vi "AskUserForModules.vi"(4 "MultiModule":bool, 6 "SkipDialog":bool, 7 "SPCModulesArray":T2[](array[typedef]) {"Bus Number" min=-1 max=255 step=1; "Base I/O Addr" format="%.0x"; "Init Status" min=-10 max=0 step=1; "in Use" min=-1 max=1 step=1; "Slot Number" min=-1 max=255 step=1; "Module Type" items=["SPC-600"=600, "SPC-630"=630, "SPC-700"=700, "SPC-730"=730, "SPC-130"=130, "SPC-830"=830, "SPC-140"=140, "SPC-930"=930, "DPC-230"=230, "SPC-150"=150, "SPC-150 N"=151, "SPC-150 NX"=152, "SPC-130 EM"=131, "SPC-130 EMN"=132, "SPC-130IN"=135, "SPC-130INX"=136, "SPC-130INXX"=137, "SPC-160"=160, "SPC-160 X"=161, "SPC-160 PCIE"=162, "SPC-180 N"=180, "SPC-180 NX"=181, "SPC-180 NXX"=182, "SPC-180 N-USB"=185, "SPC-180 NX-USB"=186, "SPC-180 NXX-USB"=187, "SPC-QC-104"=104, "SPC-QC-004"=4, "SPC-QC-106"=106, "DPC-330"=330, "PMS-800"=800, "SPC-590"=590, "Simulation"=-1]}, 8 "Error In":errorcluster={"Status"=FALSE, "Code"=0, "Source"="no error"}, 9 "Serial Number":string[](array[string]), 10 "ModuleNoArray":i16[](array[numeric]), 11 "DLL Path":path=path "C:/Program Files (x86)/BH/SPCM/DLL/spcm64.dll") -> (0 "Error Out":errorcluster, 1 "ActiveSerialNumbers":string[](array[string]), 2 "ModuleListboxStrings":string[][](array[string]), 3 "DLL Path":path=path "C:/Program Files (x86)/BH/SPCM/DLL/spcm64.dll", 5 "ActiveModuleNo":i16[](array[numeric]))   [LabVIEW 2023]
doc: "This VI presents the user with a dialog displaying all available modules with type and serial number information.\nOne or several modules can be chosen to continue with the application flow.\nThe dialog can be skipped if only one module is present or the choice already known.\nThe input values are provided by the Initialize.vi.\n\ninfo@becker-hickl.com"
uses:
  SPC_Wrappers/SPC_Controls/SPCModInfo.ctl
  SPC_Wrappers/SPC_Controls/ModuleType.ctl
panel:
  in  "Active":T1
  out "ActiveNameOfModules":string[](array[string])
  out "Module Type":string[](array[string])
  out "Name of Modules":string[](array[string])
  in  "OK":bool
  in  "Activate All":bool
  in  "Frame":string
  # "Please Choose Your TCSPC Module(s)"
  # "Developer: Frank Quadt, M.sc\n\n42 is the answer for everything!"
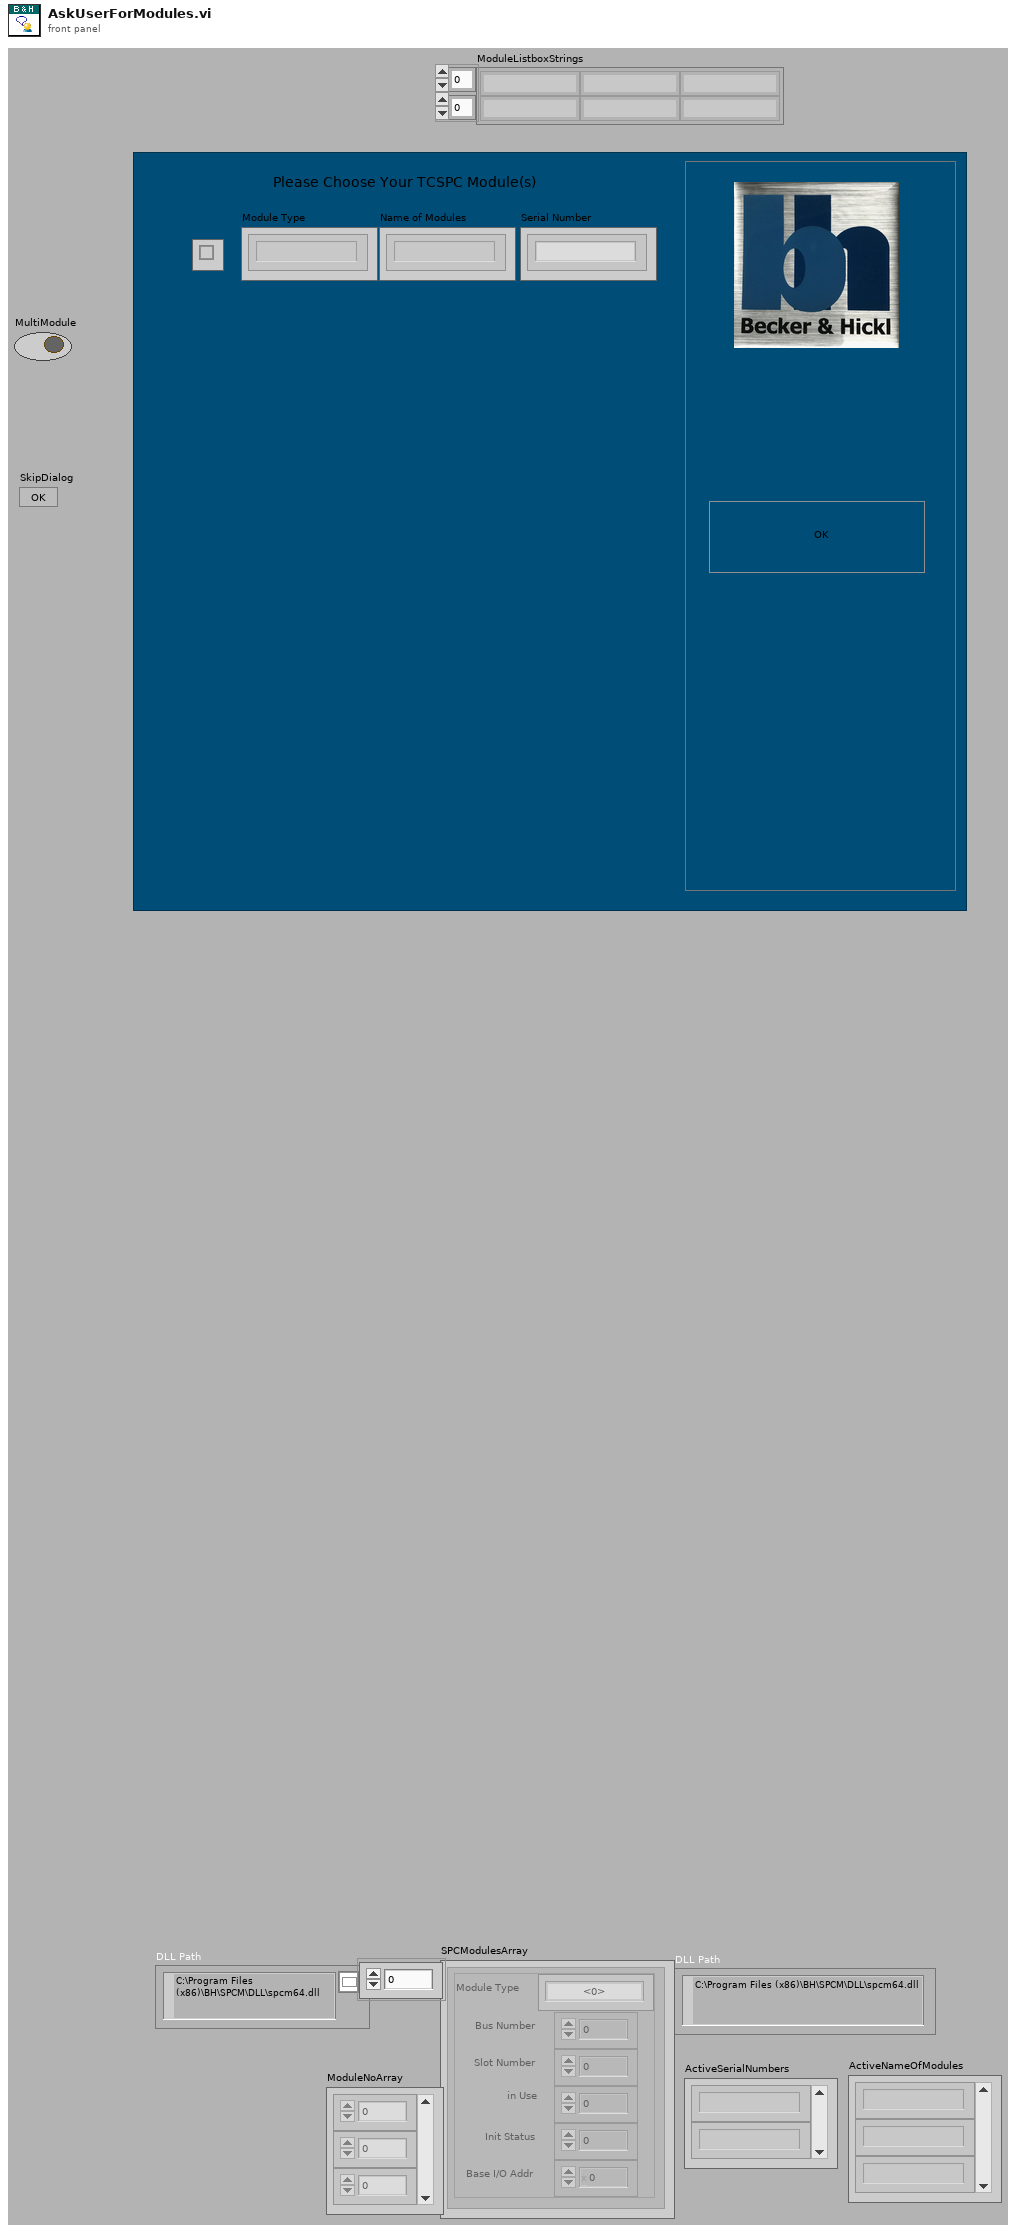
[diagram p1: front panel]
types:
  T1 = cluster{"Boolean 39":bool, "Boolean 40":bool, "Boolean 41":bool, "Boolean 42":bool, "Boolean 43":bool, "Boolean 44":bool, "Boolean 45":bool, "Boolean 46":bool, "Boolean 32":bool, "Boolean 31":bool, "Boolean 33":bool, "Boolean 34":bool, "Boolean 35":bool, "Boolean 36":bool, "Boolean 37":bool, "Boolean 38":bool, "Boolean 54":bool, "Boolean 53":bool, "Boolean 52":bool, "Boolean 51":bool, "Boolean 50":bool, "Boolean 49":bool, "Boolean 48":bool, "Boolean 47":bool, "Boolean 62":bool, "Boolean 61":bool, "Boolean 60":bool, "Boolean 59":bool, "Boolean 58":bool, "Boolean 57":bool, "Boolean 56":bool, "Boolean 55":bool}
  T2 = typedef "SPCModInfo.ctl" = cluster{"Module Type":T3, "Bus Number":i16, "Slot Number":i16, "in Use":i16, "Init Status":i16, "Base I/O Addr":u16}
  T3 = typedef "ModuleType.ctl" = i16
  T4 = enum32{"Invalid", "Default", "Floating", "Floating/Auto-Hide", "Modal"}
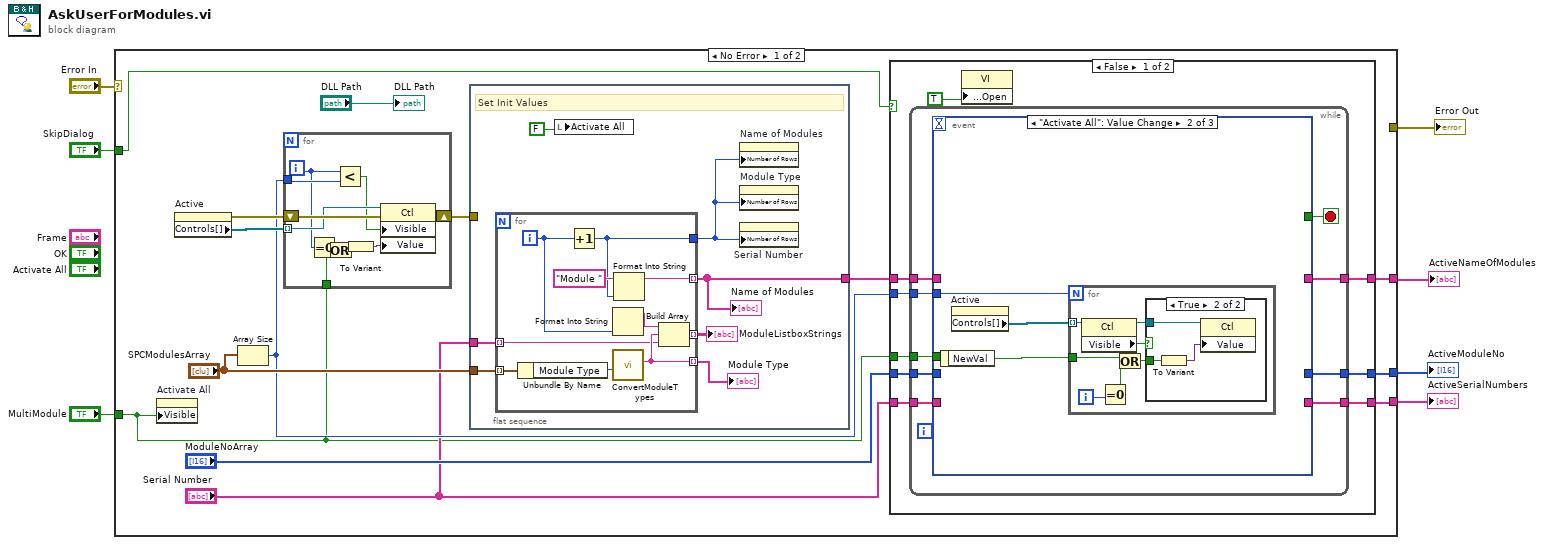
[diagram p0: block diagram]
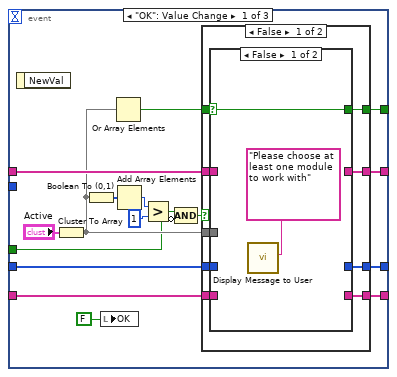
[diagram p2: hidden frame]
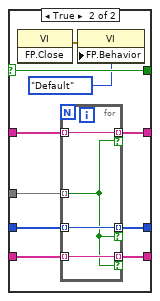
[diagram p3: hidden frame]
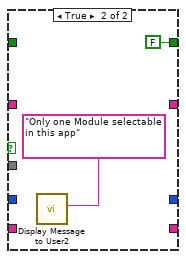
[diagram p4: hidden frame]
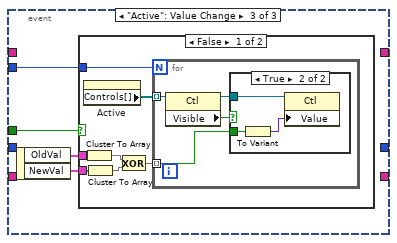
[diagram p6: hidden frame]
diagram:
  n1 = case shown="No Error" "Error In" {
    selector: "Error In" -> [_ w145]
    tunnel: [_ w145] -> w7
    tunnel: [w16 _] -> w6
    tunnel: [w15 _] -> w5
    tunnel: [w14 _] -> w4
    tunnel: "SkipDialog" -> [w9 _]
    tunnel: "MultiModule" -> [w8 _]
    frame No Error {
      n2 = property on="Activate All" class="Bool (strict)"("Visible"=w8) -> ()  [unwired: 2 in, 2 out]
      n3 = property on="Active" class="Clust (strict)"() -> (error out=w21:errorcluster, "Controls[]"=w20:refnum<vi>[])  [unwired: 2 in, 1 out]
      n4 = Array Size(array="SPCModulesArray") -> (size(s)=w11:i32)
      n5 = for {
        tunnel: w20 -> [w141] mode=indexing
        shift-right: [w144] -> w18
        shift-left: w21 -> [w143]
        tunnel: w11 -> [w140]
        tunnel: w8 -> [w135]
        i -> [w137]
        n6 = Equal To 0?(x=w137) -> (x = 0?=w138:bool)
        n7 = Or(x=w138, y=w135) -> (x .or. y?=w136:bool)
        n8 = Less?(x=w137, y=w140) -> (x < y?=w139:bool)
        n9 = To Variant(anything=w136) -> (Variant=w142:variant)
        n10 = property class="Ctl"(reference=w141, error in=w143, "Visible"=w139, "Value"=w142) -> (error out=w144:errorcluster)  [unwired: 1 out]
      }
      n11 = flat-sequence {
        tunnel: w18 -> [_]
        tunnel: [w123] -> w17
        tunnel: "SPCModulesArray" -> [w120]
        tunnel: "Serial Number" -> [w119]
        frame #0 {
          # "Set Init Values"
          n12 = for {
            tunnel: w120 -> [w134] mode=indexing
            tunnel: [w128] -> w124 mode=indexing
            tunnel: [w132] -> w123 mode=indexing
            tunnel: [w130] -> w122
            tunnel: w119 -> [w127] mode=indexing
            tunnel: [w126] -> w118 mode=indexing
            i -> [w125]
            # "Which module type matches with the production no.?"
            n13 = Unbundle By Name(w134) -> ("Module Type"=w131:T3)
            n14 = Increment(x=w125) -> (x+1=w130:i32)
            n15 = Format Into String(w125) -> (resulting string=w129:string)  [unwired: 3 in, 1 out]
            n16 = call "ConvertModuleTypes.vi"("Module TypeIn"=w131) -> ("ModuleTypeString"=w128:string)  [unwired: 8 in, 2 out]
            n17 = Format Into String(initial string="Module " ("String"), w130) -> (resulting string=w132:string)  [unwired: 2 in, 1 out]
            n18 = Build Array(w129, w128, w127) -> (w126:string[])
          }
          "Module Type" <- w124
          "Name of Modules" <- w123
          "ModuleListboxStrings" <- w118
          n19 = local write "Activate All"(FALSE) -> ()
          n20 = property on="Name of Modules" class="Arr (strict)"("Number of Rows"=w122) -> ()  [unwired: 2 in, 2 out]
          n21 = property on="Module Type" class="Arr (strict)"("Number of Rows"=w122) -> ()  [unwired: 2 in, 2 out]
          n22 = property on="Serial Number" class="Arr (strict)"("Number of Rows"=w122) -> ()  [unwired: 2 in, 2 out]
        }
      }
      n23 = case shown="False" w9 {
        tunnel: w17 -> [w30 w117]
        tunnel: [w29 w115] -> w16
        tunnel: [w28 w117] -> w15
        tunnel: [w27 w116] -> w14
        tunnel: "ModuleNoArray" -> [w26 w116]
        tunnel: w11 -> [w25 _]
        tunnel: "Serial Number" -> [w24 w115]
        tunnel: w8 -> [w22 _]
        frame False {
          n24 = while {
            tunnel: w25 -> [w38]
            tunnel: w24 -> [w36]
            tunnel: [w37] -> w29
            tunnel: [w34] -> w28
            tunnel: w30 -> [w39]
            tunnel: [w33] -> w27
            tunnel: w26 -> [w32]
            tunnel: w22 -> [w31]
            stop <- w35 stop-if-true
            n25 = event shown="[1] \"Activate All\": Value Change" {
              selector: _ -> [_ _ _]
              dyn-events: _ -> [_ _ _]
              timeout: _ -> [_ _ _]
              tunnel: w39 -> [w51 _ _]
              tunnel: [w55 _ _] -> w35
              tunnel: w38 -> [_ w86 w100]
              tunnel: [w54 _ _] -> w37
              tunnel: w36 -> [w53 _ _]
              tunnel: [w50 _ _] -> w34
              tunnel: [w49 _ _] -> w33
              tunnel: w32 -> [w48 _ _]
              tunnel: w31 -> [w41 _ w97]
              event "OK": Value Change {
                n26 = event-data() -> ()  [unwired: 1 in, 1 out]
                n27 = Cluster To Array(cluster="Active") -> (array=w46:bool[])
                n28 = Boolean To (0,1)(Boolean=w46) -> (0, 1=w45:i16[])
                n29 = local write "OK"(FALSE ("OK")) -> ()
                n30 = Or Array Elements(Boolean array=w46) -> (logical OR=w56:bool)
                n31 = Add Array Elements(numeric array=w45) -> (sum=w44:i16)
                n32 = Greater?(x=w44, y=i16 1 ("x")) -> (0:w43:bool)
                n33 = Compound Arithmetic op=AND(w43, invert w41) -> (w40:bool)
                n34 = case shown="False" w40 {
                  tunnel: w56 -> [w65 _]
                  tunnel: [w64 FALSE] -> w55
                  tunnel: [w63 _] -> w54
                  tunnel: w53 -> [w62 _]
                  tunnel: w51 -> [w61 _]
                  tunnel: [w60 _] -> w50
                  tunnel: [w59 _] -> w49
                  tunnel: w48 -> [w58 _]
                  tunnel: w46 -> [w57 _]
                  frame False {
                    n35 = case shown="False" w65 {
                      selector: w65 -> [w67 w77]
                      tunnel: [w67 w77] -> w64
                      tunnel: w57 -> [_ w76]
                      tunnel: [_ w75] -> w63
                      tunnel: w62 -> [_ w74]
                      tunnel: w61 -> [_ w73]
                      tunnel: [_ w72] -> w60
                      tunnel: [_ w71] -> w59
                      tunnel: w58 -> [_ w70]
                      frame False {
                        n36 = call "Display Message to User"("Message"="Please choose at least one module to work with") -> ()  [unwired: 9 in, 2 out]
                      }
                      frame True {
                        n37 = invoke class="VI" method="FP.Close"() -> (error out=w69:errorcluster)  [unwired: 3 in, 2 out]
                        n38 = for {
                          tunnel: w76 -> [w78] mode=indexing
                          tunnel: [w81] -> w71 mode=indexing if=w78
                          tunnel: w70 -> [w81] mode=indexing
                          tunnel: w74 -> [w80] mode=indexing
                          tunnel: [w80] -> w75 mode=indexing if=w78
                          tunnel: [w79] -> w72 mode=indexing if=w78
                          tunnel: w73 -> [w79] mode=indexing
                        }
                        n39 = property class="VI"(error in=w69, "FP.Behavior"=T4."Default" ("Front Panel Window:Behavior")) -> ()  [unwired: 1 in, 2 out]
                      }
                    }
                  }
                  frame True {
                    n40 = call "Display Message to User2"("Message"="Only one Module selectable in this app") -> ()  [unwired: 9 in, 2 out]
                  }
                }
              }
              event "Activate All": Value Change {
                n41 = event-data() -> ("NewVal"=w84:bool)  [unwired: 1 in]
                n42 = property on="Active" class="Clust (strict)"() -> ("Controls[]"=w85:refnum<vi>[])  [unwired: 2 in, 2 out]
                n43 = for {
                  N: w86 -> [_]
                  tunnel: w85 -> [w92] mode=indexing
                  tunnel: w84 -> [w93]
                  i -> [w89]
                  n44 = property class="Ctl"(reference=w92) -> (reference out=w91:refnum<vi>, "Visible"=w90:bool)  [unwired: 1 in, 1 out]
                  n45 = Equal To 0?(x=w89) -> (x = 0?=w87:bool)
                  n46 = Or(x=w93, y=w87) -> (x .or. y?=w88:bool)
                  n47 = case shown="True" w90 {
                    tunnel: w91 -> [_ w96]
                    tunnel: w88 -> [_ w94]
                    frame False {
                    }
                    frame True {
                      n48 = To Variant(anything=w94) -> (Variant=w95:variant)
                      n49 = property class="Ctl"(reference=w96, "Value"=w95) -> ()  [unwired: 1 in, 2 out]
                    }
                  }
                }
              }
              event "Active": Value Change {
                n50 = event-data() -> ("OldVal"=w99:T1, "NewVal"=w98:T1)  [unwired: 1 in]
                n51 = case shown="False" w97 {
                  tunnel: w100 -> [w107 _]
                  tunnel: w99 -> [w105 _]
                  tunnel: w98 -> [w103 _]
                  frame False {
                    n52 = property on="Active" class="Clust (strict)"() -> ("Controls[]"=w106:refnum<vi>[])  [unwired: 2 in, 2 out]
                    n53 = Cluster To Array(cluster=w105) -> (array=w102:bool[])
                    n54 = Cluster To Array(cluster=w103) -> (array=w101:bool[])
                    n55 = Exclusive Or(1:w101, 2:w102) -> (0:w104:bool[])
                    n56 = for {
                      N: w107 -> [_]
                      tunnel: w106 -> [w110] mode=indexing
                      tunnel: w104 -> [w111] mode=indexing
                      n57 = property class="Ctl"(reference=w110) -> (reference out=w109:refnum<vi>, "Visible"=w108:bool)  [unwired: 1 in, 1 out]
                      n58 = case shown="True" w108 {
                        tunnel: w109 -> [_ w114]
                        tunnel: w111 -> [_ w112]
                        frame False {
                        }
                        frame True {
                          n59 = To Variant(anything=w112) -> (Variant=w113:variant)
                          n60 = property class="Ctl"(reference=w114, "Value"=w113) -> ()  [unwired: 1 in, 2 out]
                        }
                      }
                    }
                  }
                  frame True {
                  }
                }
              }
            }
          }
          n61 = property class="VI"("Front Panel Window:Open"=TRUE) -> ()  [unwired: 2 in, 2 out]
        }
        frame True {
        }
      }
      "DLL Path" <- "DLL Path"
    }
    frame Error {
    }
  }
  "Error Out" <- w7
  "ActiveSerialNumbers" <- w6
  "ActiveNameOfModules" <- w5
  "ActiveModuleNo" <- w4
